vi "Create TestCase Template Instance_rcf.vi"(8 "error in":errorcluster, 11 "Application Ref (This Application)":refnum<vi>) -> (0 "error out":errorcluster, 3 "Application Ref":refnum<vi>)   [LabVIEW 2009]
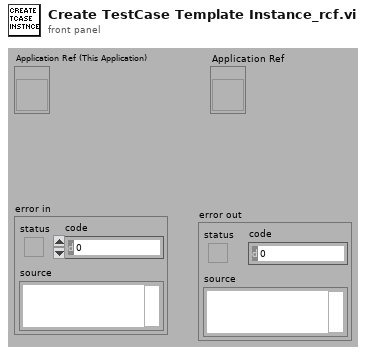
[diagram p1: front panel]
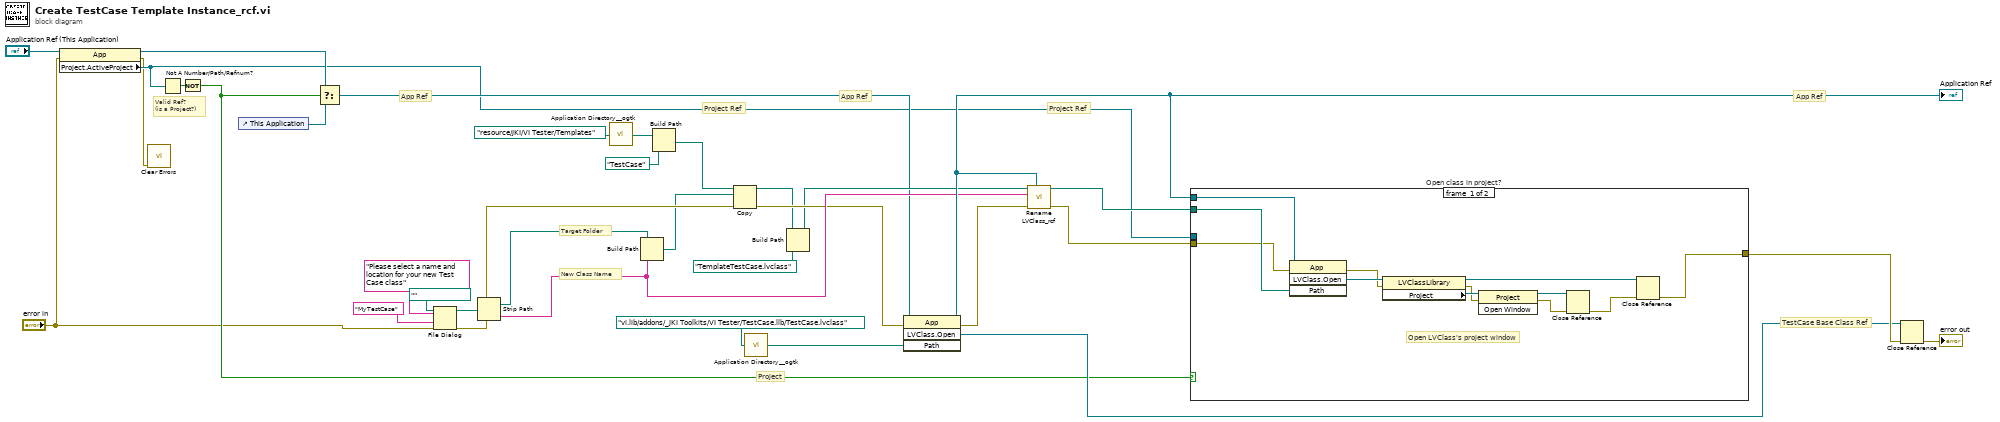
[diagram p0: block diagram]
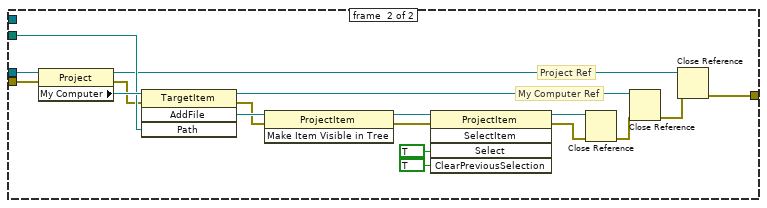
[diagram p2: hidden frame]
diagram:
  # "Project Ref"
  # "App Ref"
  # "Valid Ref?\n(is a Project?)"
  # "TestCase Base Class Ref"
  # "Project"
  # "App Ref"
  # "Project Ref"
  # "App Ref"
  # "Target Folder"
  # "New Class Name"
  n1 = property class="App"(reference="Application Ref (This Application)", error in="error in") -> (reference out=w7:refnum<vi>, error out=w2:errorcluster, "Project.ActiveProject"=w3:refnum<vi>)
  n2 = call <vilib>:"Clear Errors.vi"("error in (no error)"=w2) -> ()  [unwired: 6 in, 1 out]
  n3 = Not A Number/Path/Refnum?(number/path/refnum=w3) -> (NaN/Path/Refnum?=w9:bool)
  n4 = Not(x=w9) -> (.not. x?=w4:bool)
  n5 = control-ref of="This Application"() -> (w8:refnum<vi>)
  n6 = Select(t=w7, s=w4, f=w8) -> (s? t:f=w5:refnum<vi>)
  n7 = File Dialog(7:"Please select a name and location for your new Test Case class" ("prompt"), 8:"error in", 9:"MyTestCase" ("default name"), 11:path "" ("start path")) -> (0:w34:errorcluster, 3:w33:path)  [unwired: 3 in, 2 out]
  n8 = Strip Path(path=w33) -> (stripped path=w24:path, name=w25:string)
  n9 = call <userlib>:"Application Directory__ogtk.vi"("Relative path (.)"=path "resource/JKI/VI Tester/Templates") -> ("Application Directory (+ Relative)"=w11:path)
  n10 = Build Path(base path=w24, name or relative path=w25) -> (appended path=w14:path)
  n11 = Build Path(base path=w11, name or relative path=path "TestCase") -> (appended path=w13:path)
  n12 = Copy(8:w34, 10:w14, 11:w13) -> (0:w20:errorcluster, 3:w15:path)  [unwired: 2 in, 1 out]
  n13 = call <userlib>:"Application Directory__ogtk.vi"("Relative path (.)"=path "vi.lib/addons/_JKI Toolkits/VI Tester/TestCase.llb/TestCase.lvclass") -> ("Application Directory (+ Relative)"=w19:path)
  n14 = Build Path(base path=w15, name or relative path=path "TemplateTestCase.lvclass") -> (appended path=w17:path)
  n15 = invoke class="App" method="LVClass.Open"(reference=w5, error in=w20, "Path"=w19) -> (reference out=w31:refnum<vi>, error out=w21:errorcluster, "LVClass.Open"=w28:refnum<vi>)  [unwired: 1 in, 1 out]
  "Application Ref" <- w31
  n16 = call "Rename LVClass_rcf.vi"("App reference"=w31, "error in (no error)"=w21, "New Class Name"=w25, "LVClass Path"=w17) -> ("error out"=w27:errorcluster, "Updated LVClass Path"=w26:path)  [unwired: 6 in]
  n17 = case "Open class in project?" shown="False" w4 {
    tunnel: w26 -> [w44 w63]
    tunnel: w27 -> [w43 w61]
    tunnel: [w41 w56] -> w30
    tunnel: w3 -> [_ w47]
    tunnel: w31 -> [w37 _]
    frame #0 {
      # "Open LVClass's project window"
      n18 = invoke class="App" method="LVClass.Open"(reference=w37, error in=w43, "Path"=w44) -> (error out=w45:errorcluster, "LVClass.Open"=w46:refnum<vi>)  [unwired: 1 in, 2 out]
      n19 = property class="LVClassLibrary"(reference=w46, error in=w45) -> (reference out=w42:refnum<vi>, error out=w39:errorcluster, "Project"=w40:refnum<vi>)
      n20 = invoke class="Project" method="Open Window"(reference=w40, error in=w39) -> (reference out=w38:refnum<vi>, error out=w36:errorcluster)  [unwired: 1 in, 1 out]
      n21 = Close Reference(reference=w38, error in (no error)=w36) -> (error out=w35:errorcluster)
      n22 = Close Reference(reference=w42, error in (no error)=w35) -> (error out=w41:errorcluster)
    }
    frame #1 {
      # "My Computer Ref"
      # "Project Ref"
      n23 = property class="Project"(reference=w47, error in=w61) -> (reference out=w58:refnum<vi>, error out=w62:errorcluster, "My Computer"=w64:refnum<vi>)
      n24 = invoke class="TargetItem" method="AddFile"(reference=w64, error in=w62, "Path"=w63) -> (reference out=w59:refnum<vi>, error out=w54:errorcluster, "AddFile"=w55:refnum<vi>)  [unwired: 1 in, 1 out]
      n25 = invoke class="ProjectItem" method="Make Item Visible in Tree"(reference=w55, error in=w54) -> (reference out=w51:refnum<vi>, error out=w53:errorcluster)  [unwired: 1 in, 1 out]
      n26 = invoke class="ProjectItem" method="SelectItem"(reference=w51, error in=w53, "Select"=TRUE, "ClearPreviousSelection"=TRUE) -> (reference out=w50:refnum<vi>, error out=w52:errorcluster)  [unwired: 1 in, 3 out]
      n27 = Close Reference(reference=w50, error in (no error)=w52) -> (error out=w60:errorcluster)
      n28 = Close Reference(reference=w59, error in (no error)=w60) -> (error out=w57:errorcluster)
      n29 = Close Reference(reference=w58, error in (no error)=w57) -> (error out=w56:errorcluster)
    }
  }
  n30 = Close Reference(reference=w28, error in (no error)=w30) -> (error out=→"error out":errorcluster)
